vi "Read Sample Temperature.vi"(0 "VISA Refnum in":refnum<visa-resource-name>, 3 "error in (no error)":errorcluster) -> (7 "VISA Refnum out":refnum<visa-resource-name>, 8 "Temperature":dbl, 10 "error out":errorcluster)   [LabVIEW 2019]
uses:
  <vilib>/Utility/error.llb/Error Cluster From Error Code.vi
  <vilib>/regexp/Match Regular Expression.xnode
  <vilib>/ErrorRing/Error Ring.xnode
panel:
  out "String":string
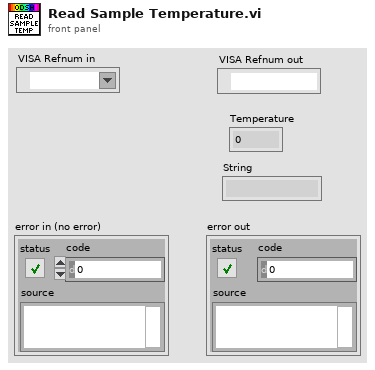
[diagram p1: front panel]
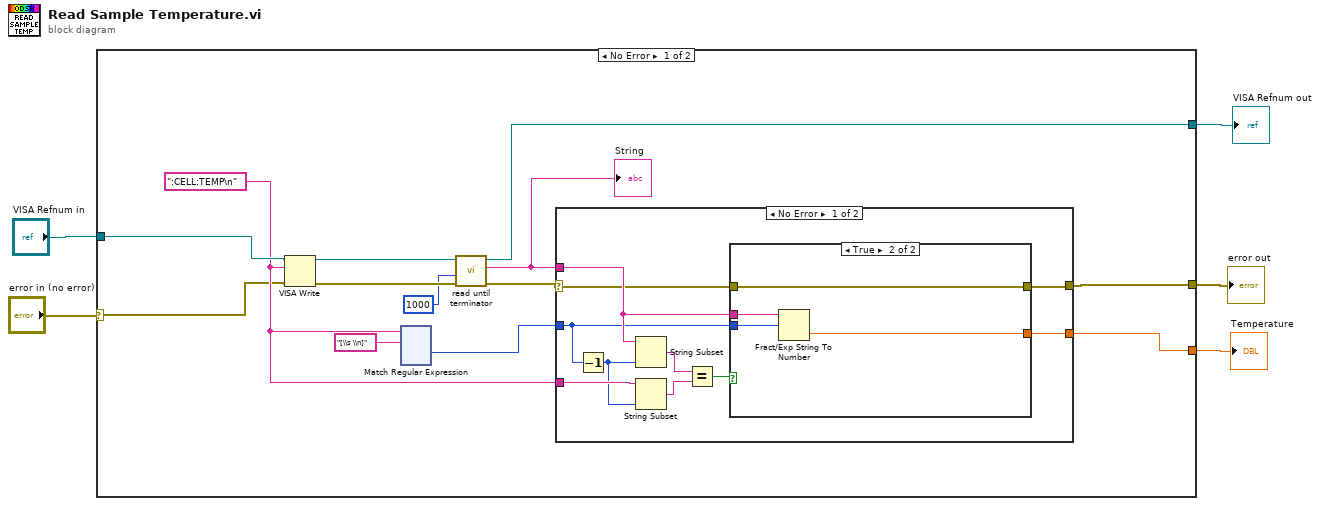
[diagram p0: block diagram]
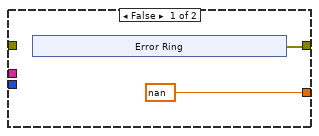
[diagram p2: hidden frame]
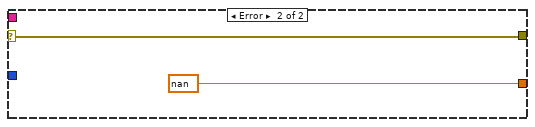
[diagram p3: hidden frame]
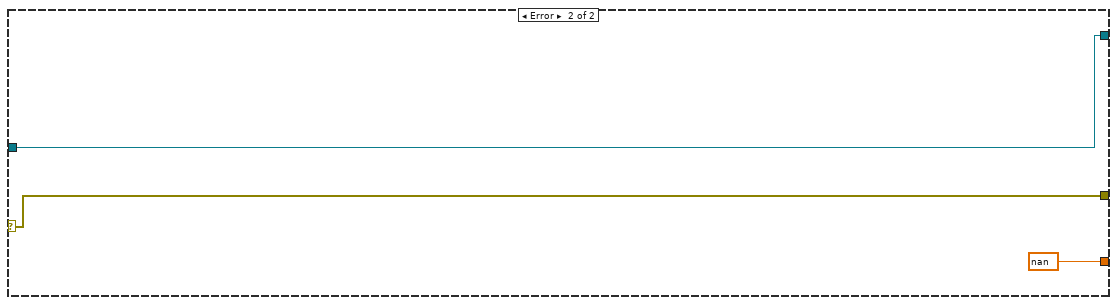
[diagram p4: hidden frame]
diagram:
  n1 = case shown="No Error" "error in (no error)" {
    selector: "error in (no error)" -> [w6 w158]
    tunnel: "VISA Refnum in" -> [w18 w157]
    tunnel: [w15 w157] -> w4
    tunnel: [w13 nan] -> w3
    tunnel: [w11 w158] -> w2
    frame No Error {
      w7 = ":CELL:TEMP\n" ("buffer d'écriture")
      n2 = VISA Write(VISA resource name=w18, write buffer=w7, error in (no error)=w6) -> (VISA resource name out=w17:refnum<visa-resource-name>, error out=w16:errorcluster)  [unwired: 1 out]
      n3 = xnode "Match Regular Expression"("input string"=w7, "regular expression"="[\\s \\n]") -> ("offset past match"=w8:i32)  [unwired: 4 in, 4 out]
      n4 = call "read until terminator.vi"("error in (no error)"=w16, "Timeout (ms)"=1000, "VISA Refnum in"=w17) -> ("error out"=w12:errorcluster, "String"=w10:string, "VISA Refnum out"=w15:refnum<visa-resource-name>)  [unwired: 6 in]
      "String" <- w10
      n5 = case shown="No Error" w12 {
        selector: w12 -> [w136 w154]
        tunnel: w10 -> [w140 _]
        tunnel: [w142 nan] -> w13
        tunnel: [w135 w154] -> w11
        tunnel: w8 -> [w134 _]
        tunnel: w7 -> [w141 _]
        frame No Error {
          n6 = Decrement(x=w134) -> (x-1=w133:i32)
          n7 = String Subset(string=w140, length (rest)=w133) -> (substring=w139:string)  [unwired: 1 in]
          n8 = String Subset(string=w141, length (rest)=w133) -> (substring=w138:string)  [unwired: 1 in]
          n9 = Equal?(x=w139, y=w138) -> (x = y?=w137:bool)
          n10 = case shown="True" w137 {
            tunnel: [nan w153] -> w142
            tunnel: w140 -> [_ w152]
            tunnel: w134 -> [_ w151]
            tunnel: w136 -> [_ w150]
            tunnel: [w143 w150] -> w135
            frame False {
              n11 = xnode "Error Ring"() -> ("error out"=w143:errorcluster)
            }
            frame True {
              n12 = Fract/Exp String To Number(string=w152, offset=w151) -> (number=w153:dbl)  [unwired: 2 in, 1 out]
            }
          }
        }
        frame Error {
        }
      }
    }
    frame Error {
    }
  }
  "error out" <- w2
  "VISA Refnum out" <- w4
  "Temperature" <- w3
